vi "bigcryo-T-full_step.vi"() -> (2 "VTI [K]":dbl=99.5, 3 "Spl [K]":dbl=292.757)   [LabVIEW 2019]
uses:
  Components/Global 2.vi
  <vilib>/Analysis/NI_AALPro.lvlib
panel:
  out "Exec T":u32=289
  out "Stable?":bool
  in  "stop":bool
  out "Running Sequence":bool
  out "VTI Rate":dbl=-0.0022185709228587803 format="%#.3g"
  out "Rate":dbl=-0.05046918842629548 format="%#.3g"
  in  "Rate":dbl=0.5
  in  "Reset Graph":bool
  in  "Ramp":bool
  in  "Go To":bool
  in  "Set Temp":dbl=100.0
  out "Range":dbl=5.0
  out "Spl":dbl(slide) scale=0.0..100.0
  out "VTI":dbl(slide)=5.7 scale=0.0..100.0
  out "T":cluster{"X":dbl[], "Y":dbl[]}[](graph)=[{"X"=[16.312679499999998, 16.601001399999998, 16.8885939, 17.146738, 17.4184414, 17.704434499999998, 17.976812, 18.2486923, 18.519247699999998, 18.8086779, 19.0817953, 19.3520784, 19.6253158, 19.913267299999998, 20.186597499999998, 20.457057199999998, 20.7287552, 21.0156451, 21.2713833, 21.5449196, 21.834149999999998, 22.1212511, 22.375041, 22.6487737, 22.93645, 23.2227294, 23.47921, 23.751889799999997, 24.0381173, 24.3104694, 24.5817102, 24.8549242, 25.1436846, 25.4137649, 25.6865617, 25.9587959, 26.2467246, 26.519138299999998, 26.788798399999997, 27.0636323, 27.351064299999997, 27.6211639, 27.894986399999997, 28.1650033, 28.4524293, 28.7077293, 28.981569999999998, 29.2689606, 29.5564118, 29.8125924, 30.0829135, 30.3731589, 30.6605563, 30.9164724, 31.1880325, 31.476441299999998, 31.7628693, 32.0191987, 32.291540399999995, 32.581536899999996, 32.8666054, 33.123576199999995, 33.393609399999995, 33.6835326, 33.9546916, 34.2266786, 34.5016617, 34.7865946, 35.0595013, 35.3305311, 35.6012708, 35.8907765, 36.1449745, 36.4181133, 36.7055869, 36.9932881, 37.2491099, 37.5211332, 37.8092405, 38.096976999999995, 38.3524566, 38.6252108, 38.9137998, 39.202196099999995, 39.4708979, 39.7266816, 40.0164993, 40.2877493, 40.5591022, 40.8298363, 41.1201748, 41.392564, 41.6641809, 41.935850699999996, 42.224531999999996, 42.493339299999995, 42.767248699999996, 43.0566812, 43.341667699999995, 43.6315349, 43.9040886, 44.1748267, 44.461991399999995, 44.7503789, 45.0366612, 45.292437799999995, 45.5670358, 45.8529609, 46.1413034, 46.397208199999994, 46.6697953, 46.955648, 47.2436574, 47.50036, 47.773001099999995, 48.060690199999996, 48.347202599999996, 48.6065446, 48.8750785, 49.1640923, 49.4524638, 49.708949, 49.9802385, 50.266528199999996, 50.5407401, 50.812329999999996, 51.0825536], "Y"=[99.498, 99.498, 99.498, 99.498, 99.498, 99.499, 99.499, 99.499, 99.5, 99.5, 99.5, 99.5, 99.5, 99.5, 99.5, 99.501, 99.501, 99.5, 99.5, 99.501, 99.5, 99.501, 99.501, 99.501, 99.501, 99.501, 99.501, 99.501, 99.501, 99.501, 99.501, 99.5, 99.5, 99.5, 99.5, 99.5, 99.501, 99.501, 99.502, 99.502, 99.502, 99.503, 99.502, 99.503, 99.503, 99.502, 99.502, 99.501, 99.501, 99.501, 99.501, 99.5, 99.499, 99.499, 99.499, 99.499, 99.5, 99.501, 99.501, 99.501, 99.501, 99.5, 99.5, 99.5, 99.501, 99.501, 99.501, 99.501, 99.501, 99.501, 99.5, 99.5, 99.5, 99.5, 99.501, 99.501, 99.501, 99.5, 99.5, 99.5, 99.501, 99.5, 99.5, 99.499, 99.499, 99.499, 99.499, 99.499, 99.499, 99.499, 99.5, 99.499, 99.499, 99.499, 99.499, 99.5, 99.5, 99.5, 99.5, 99.5, 99.5, 99.5, 99.5, 99.501, 99.5, 99.501, 99.5, 99.5, 99.501, 99.5, 99.501, 99.501, 99.502, 99.501, 99.501, 99.501, 99.501, 99.5, 99.501, 99.5, 99.5, 99.5, 99.5, 99.5, 99.499, 99.499, 99.5]}, {"X"=[16.312679499999998, 16.601001399999998, 16.8885939, 17.146738, 17.4184414, 17.704434499999998, 17.976812, 18.2486923, 18.519247699999998, 18.8086779, 19.0817953, 19.3520784, 19.6253158, 19.913267299999998, 20.186597499999998, 20.457057199999998, 20.7287552, 21.0156451, 21.2713833, 21.5449196, 21.834149999999998, 22.1212511, 22.375041, 22.6487737, 22.93645, 23.2227294, 23.47921, 23.751889799999997, 24.0381173, 24.3104694, 24.5817102, 24.8549242, 25.1436846, 25.4137649, 25.6865617, 25.9587959, 26.2467246, 26.519138299999998, 26.788798399999997, 27.0636323, 27.351064299999997, 27.6211639, 27.894986399999997, 28.1650033, 28.4524293, 28.7077293, 28.981569999999998, 29.2689606, 29.5564118, 29.8125924, 30.0829135, 30.3731589, 30.6605563, 30.9164724, 31.1880325, 31.476441299999998, 31.7628693, 32.0191987, 32.291540399999995, 32.581536899999996, 32.8666054, 33.123576199999995, 33.393609399999995, 33.6835326, 33.9546916, 34.2266786, 34.5016617, 34.7865946, 35.0595013, 35.3305311, 35.6012708, 35.8907765, 36.1449745, 36.4181133, 36.7055869, 36.9932881, 37.2491099, 37.5211332, 37.8092405, 38.096976999999995, 38.3524566, 38.6252108, 38.9137998, 39.202196099999995, 39.4708979, 39.7266816, 40.0164993, 40.2877493, 40.5591022, 40.8298363, 41.1201748, 41.392564, 41.6641809, 41.935850699999996, 42.224531999999996, 42.493339299999995, 42.767248699999996, 43.0566812, 43.341667699999995, 43.6315349, 43.9040886, 44.1748267, 44.461991399999995, 44.7503789, 45.0366612, 45.292437799999995, 45.5670358, 45.8529609, 46.1413034, 46.397208199999994, 46.6697953, 46.955648, 47.2436574, 47.50036, 47.773001099999995, 48.060690199999996, 48.347202599999996, 48.6065446, 48.8750785, 49.1640923, 49.4524638, 49.708949, 49.9802385, 50.266528199999996, 50.5407401, 50.812329999999996, 51.0825536], "Y"=[292.743, 292.755, 292.765, 292.763, 292.773, 292.772, 292.766, 292.779, 292.785, 292.778, 292.764, 292.754, 292.748, 292.753, 292.754, 292.771, 292.771, 292.764, 292.753, 292.757, 292.751, 292.75, 292.763, 292.761, 292.764, 292.763, 292.768, 292.761, 292.761, 292.749, 292.776, 292.764, 292.769, 292.772, 292.771, 292.768, 292.772, 292.77, 292.769, 292.764, 292.773, 292.78, 292.785, 292.78, 292.761, 292.76, 292.757, 292.773, 292.779, 292.791, 292.776, 292.776, 292.783, 292.783, 292.776, 292.762, 292.767, 292.778, 292.778, 292.767, 292.765, 292.769, 292.769, 292.773, 292.768, 292.766, 292.761, 292.762, 292.737, 292.748, 292.752, 292.739, 292.739, 292.731, 292.734, 292.746, 292.733, 292.732, 292.727, 292.736, 292.742, 292.736, 292.735, 292.747, 292.766, 292.768, 292.755, 292.749, 292.768, 292.761, 292.772, 292.759, 292.756, 292.759, 292.753, 292.747, 292.751, 292.742, 292.738, 292.746, 292.745, 292.743, 292.744, 292.737, 292.745, 292.757, 292.756, 292.769, 292.753, 292.757, 292.75, 292.751, 292.74, 292.737, 292.748, 292.758, 292.765, 292.765, 292.761, 292.759, 292.757, 292.756, 292.757, 292.754, 292.759, 292.763, 292.757]}] caption="XY Graph"
  out "Set VTI [K]":dbl=99.5
  out "Set Spl [K]":dbl=100.0
  # "Heaters"
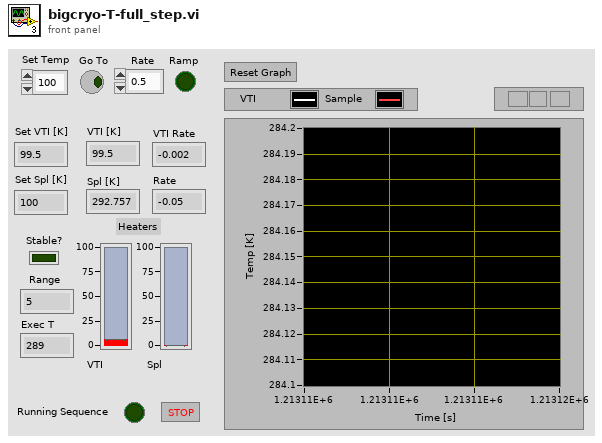
[diagram p1: front panel]
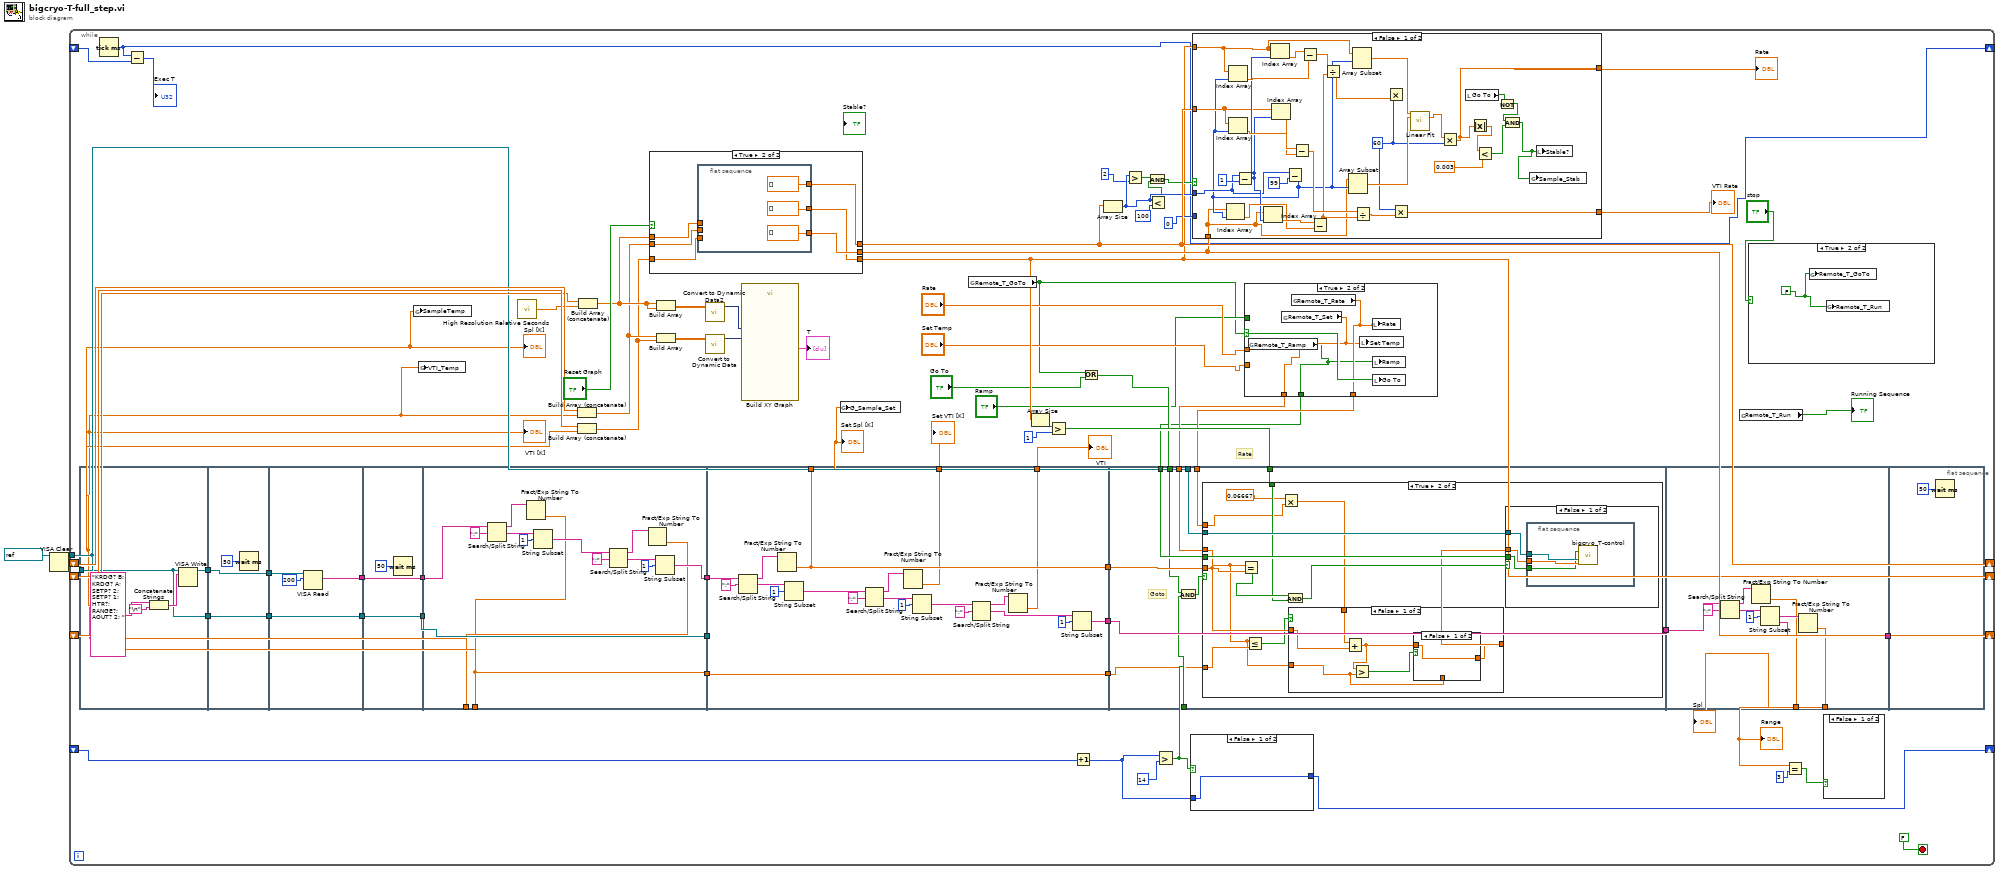
[diagram p0: block diagram]
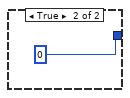
[diagram p2: hidden frame]
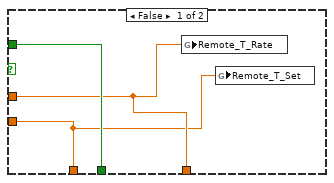
[diagram p4: hidden frame]
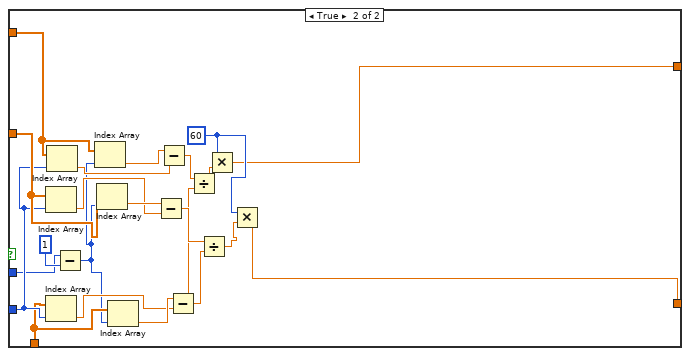
[diagram p5: hidden frame]
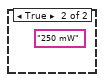
[diagram p7: hidden frame]
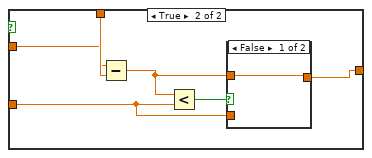
[diagram p10: hidden frame]
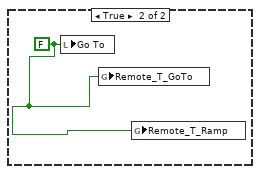
[diagram p12: hidden frame]
diagram:
  n1 = VISA Clear(VISA resource name=refnum<visa-resource-name> "COM7" ("Lakeshore Address")) -> (VISA resource name out=w2:refnum<visa-resource-name>)  [unwired: 1 in, 1 out]
  n2 = while {
    tunnel: w2 -> [w44]
    shift-right: [w29] -> _
    shift-left: _ -> [w72]
    shift-right: [w41] -> _
    shift-left: _ -> [w71]
    shift-right: [w38] -> _
    shift-left: _ -> [w69]
    shift-right: [w15] -> _
    shift-left: _ -> [w17]
    shift-right: [w11] -> _
    shift-left: _ -> [w10]
    stop <- FALSE stop-if-true
    # "Rate"
    n3 = flat-sequence {
      tunnel: w44 -> [w152]
      tunnel: [w152] -> w54
      tunnel: [w151] -> w51
      tunnel: w54 -> [w158]
      tunnel: [w158] -> w53
      tunnel: [w156] -> w52
      tunnel: w51 -> [w156]
      tunnel: [w162] -> w60
      tunnel: w53 -> [w162]
      tunnel: w52 -> [w160]
      tunnel: [w159] -> w48
      tunnel: [w165] -> w76
      tunnel: w60 -> [w165]
      tunnel: [w163] -> w49
      tunnel: w48 -> [w163]
      tunnel: w76 -> [w179]
      tunnel: [w167] -> w6
      tunnel: [w166] -> w7
      tunnel: [w179] -> w73
      tunnel: [w168] -> w50
      tunnel: w49 -> [w170]
      tunnel: [w166] -> w9
      tunnel: [w199] -> w46
      tunnel: [w198] -> w43
      tunnel: [w197] -> w63
      tunnel: [w191] -> w75
      tunnel: [w198] -> w3
      tunnel: w50 -> [w182]
      tunnel: w73 -> [_]
      tunnel: w9 -> [w180]
      tunnel: [w180] -> w8
      tunnel: w46 -> [w210]
      tunnel: [w210] -> w45
      tunnel: w25 -> [w202]
      tunnel: w44 -> [w209]
      tunnel: w21 -> [w208]
      tunnel: w19 -> [w207]
      tunnel: w23 -> [w206]
      tunnel: w43 -> [w205]
      tunnel: w27 -> [w204]
      tunnel: w13 -> [w203]
      tunnel: w8 -> [w200]
      tunnel: [w254] -> w47
      tunnel: [w253] -> w42
      tunnel: w45 -> [w247]
      tunnel: [w252] -> w55
      tunnel: w47 -> [_]
      frame #0 {
        n4 = Concatenate Strings("KRDG? B; KRDG? A; SETP? 2; SETP? 1; HTR?; RANGE?; AOUT? 2; " ("write buffer"), "\n") -> (w153:string)
        n5 = VISA Write(VISA resource name=w152, write buffer=w153) -> (VISA resource name out=w151:refnum<visa-resource-name>)  [unwired: 1 in, 2 out]
      }
      frame #1 {
        n6 = Wait (ms)(milliseconds to wait=50) -> ()  [unwired: 1 out]
      }
      frame #2 {
        n7 = VISA Read(VISA resource name=w160, byte count=u32 200) -> (read buffer=w159:string)  [unwired: 1 in, 3 out]
      }
      frame #3 {
        n8 = Wait (ms)(milliseconds to wait=50) -> ()  [unwired: 1 out]
      }
      frame #4 {
        n9 = Search/Split String(string=w170, search string/char (-)=";") -> (substring before match=w175:string, match + rest of string=w177:string)  [unwired: 1 in, 1 out]
        n10 = Fract/Exp String To Number(string=w175) -> (number=w166:dbl)  [unwired: 3 in, 1 out]
        n11 = String Subset(string=w177, offset (0)=u32 1 ("byte count")) -> (substring=w169:string)  [unwired: 1 in]
        n12 = Search/Split String(string=w169, search string/char (-)=";") -> (substring before match=w171:string, match + rest of string=w173:string)  [unwired: 1 in, 1 out]
        n13 = Fract/Exp String To Number(string=w171) -> (number=w167:dbl)  [unwired: 3 in, 1 out]
        n14 = String Subset(string=w173, offset (0)=u32 1 ("byte count")) -> (substring=w168:string)  [unwired: 1 in]
      }
      frame #5 {
        n15 = Search/Split String(string=w182, search string/char (-)=";") -> (substring before match=w181:string, match + rest of string=w184:string)  [unwired: 1 in, 1 out]
        n16 = Fract/Exp String To Number(string=w181) -> (number=w198:dbl)  [unwired: 3 in, 1 out]
        n17 = String Subset(string=w184, offset (0)=u32 1 ("byte count")) -> (substring=w187:string)  [unwired: 1 in]
        n18 = Search/Split String(string=w187, search string/char (-)=";") -> (substring before match=w186:string, match + rest of string=w189:string)  [unwired: 1 in, 1 out]
        n19 = Fract/Exp String To Number(string=w186) -> (number=w191:dbl)  [unwired: 3 in, 1 out]
        n20 = String Subset(string=w189, offset (0)=u32 1 ("byte count")) -> (substring=w193:string)  [unwired: 1 in]
        n21 = Search/Split String(string=w193, search string/char (-)=";") -> (substring before match=w192:string, match + rest of string=w195:string)  [unwired: 1 in, 1 out]
        n22 = Fract/Exp String To Number(string=w192) -> (number=w197:dbl)  [unwired: 3 in, 1 out]
        n23 = String Subset(string=w195, offset (0)=u32 1 ("byte count")) -> (substring=w199:string)  [unwired: 1 in]
      }
      frame #6 {
        # "Goto"
        n24 = And(x=w202, y=w203) -> (x .and. y?=w201:bool)
        n25 = case shown="True" w201 {
          tunnel: w209 -> [_ w223]
          tunnel: w208 -> [_ w211]
          tunnel: w207 -> [_ w222]
          tunnel: w206 -> [_ w217]
          tunnel: w205 -> [_ w214]
          tunnel: w204 -> [_ w220]
          tunnel: w200 -> [_ w216]
          frame False {
          }
          frame True {
            n26 = Equal?(x=w211, y=w214) -> (x = y?=w221:bool)
            n27 = Less Or Equal?(x=w211, y=w216) -> (x <= y?=w212:bool)
            n28 = Multiply(x=0.06667, y=w217) -> (x*y=w215:dbl)
            n29 = And(x=w221, y=w220) -> (x .and. y?=w219:bool)
            n30 = case shown="False" w212 {
              tunnel: w215 -> [w229 w237]
              tunnel: w214 -> [w228 w236]
              tunnel: [w224 w233] -> w213
              tunnel: w211 -> [w227 w232]
              frame False {
                n31 = Add(x=w229, y=w228) -> (x+y=w225:dbl)
                n32 = Greater?(x=w225, y=w227) -> (0:w226:bool)
                n33 = case shown="False" w226 {
                  tunnel: w227 -> [_ w231]
                  tunnel: w225 -> [w230 _]
                  tunnel: [w230 w231] -> w224
                  frame False {
                  }
                  frame True {
                  }
                }
              }
              frame True {
                n34 = Subtract(x=w236, y=w237) -> (x-y=w234:dbl)
                n35 = Less?(x=w234, y=w232) -> (x < y?=w235:bool)
                n36 = case shown="False" w235 {
                  tunnel: w234 -> [w238 _]
                  tunnel: [w238 w239] -> w233
                  tunnel: w232 -> [_ w239]
                  frame False {
                  }
                  frame True {
                  }
                }
              }
            }
            n37 = case shown="False" w219 {
              tunnel: w223 -> [w242 _]
              tunnel: w213 -> [w241 _]
              tunnel: w222 -> [w240 _]
              frame False {
                n38 = flat-sequence {
                  tunnel: w242 -> [w245]
                  tunnel: w241 -> [w244]
                  tunnel: w240 -> [w243]
                  frame #0 {
                    n39 = call "bigcryo_T-control.vi"("Ramp Mode"=w243, "VISA resource name out"=w245, "Set Sample Temp [K]"=w244) -> ()  [unwired: 13 in]
                  }
                }
              }
              frame True {
                w246 = FALSE
                n40 = local write "Go To"(w246) -> ()
                n41 = global write "Global 2.vi" "Remote_T_GoTo"(w246) -> ()
                n42 = global write "Global 2.vi" "Remote_T_Ramp"(w246) -> ()
              }
            }
          }
        }
      }
      frame #7 {
        n43 = Search/Split String(string=w247, search string/char (-)=";") -> (substring before match=w248:string, match + rest of string=w250:string)  [unwired: 1 in, 1 out]
        n44 = Fract/Exp String To Number(string=w248) -> (number=w252:dbl)  [unwired: 3 in, 1 out]
        n45 = String Subset(string=w250, offset (0)=u32 1 ("byte count")) -> (substring=w254:string)  [unwired: 1 in]
        n46 = Fract/Exp String To Number(string=w254) -> (number=w253:dbl)  [unwired: 3 in, 1 out]
      }
      frame #8 {
        n47 = Wait (ms)(milliseconds to wait=50) -> ()  [unwired: 1 out]
      }
    }
    n48 = Tick Count (ms)() -> (millisecond timer value=w15:u32)
    n49 = Subtract(x=w15, y=w17) -> (x-y=→"Exec T":u32)
    n50 = global write "Global 2.vi" "SampleTemp"(w7) -> ()
    n51 = global write "Global 2.vi" "VTI_Temp"(w6) -> ()
    n52 = call <vilib>:"High Resolution Relative Seconds.vi"() -> ("relative seconds"=w68:dbl)
    n53 = Build Array (concatenate)(w71, w6) -> (w57:dbl[])
    n54 = Build Array (concatenate)(w72, w7) -> (w56:dbl[])
    n55 = Build Array (concatenate)(w69, w68) -> (w58:dbl[])
    n56 = case shown="True" "Reset Graph" {
      tunnel: w58 -> [w141 w147]
      tunnel: [w141 w146] -> w38
      tunnel: w57 -> [w140 w145]
      tunnel: [w140 w144] -> w41
      tunnel: w56 -> [w139 w143]
      tunnel: [w139 w142] -> w29
      frame False {
      }
      frame True {
        n57 = flat-sequence {
          tunnel: w147 -> [_]
          tunnel: w145 -> [_]
          tunnel: w143 -> [_]
          tunnel: [dbl[] []] -> w144
          tunnel: [dbl[] []] -> w146
          tunnel: [dbl[] []] -> w142
          frame #0 {
          }
        }
      }
    }
    n58 = Build Array(w58, w58) -> (w65:dbl[][])
    n59 = Build Array(w57, w56) -> (w67:dbl[][])
    n60 = call "Convert to Dynamic Data2"("2D Array"=w65) -> ("Dynamic Data Type"=w64:dynamicdata)  [unwired: 3 in]
    n61 = call "Convert to Dynamic Data"("2D Array"=w67) -> ("Dynamic Data Type"=w66:dynamicdata)  [unwired: 3 in]
    n62 = call "Build XY Graph"("Y Input"=w66, "X Input"=w64) -> ("XY Graph"=→"T":cluster{"X":dbl[], "Y":dbl[]}[])  [unwired: 8 in, 1 out]
    n63 = global write "Global 2.vi" "G_Sample_Set"(w3) -> ()
    n64 = global read "Global 2.vi" "Remote_T_GoTo"() -> (w5:bool)
    n65 = Array Size(array=w29) -> (size(s)=w30:i32)
    n66 = Greater?(x=w30, y=1) -> (0:w27:bool)
    n67 = Increment(x=w10) -> (x+1=w12:i32)
    n68 = Or(x=w5, y="Go To") -> (x .or. y?=w25:bool)
    n69 = Array Size(array=w41) -> (size(s)=w35:i32)
    n70 = Greater?(x=w35, y=2) -> (0:w37:bool)
    n71 = Less?(x=w35, y=100) -> (x < y?=w33:bool)
    n72 = And(x=w37, y=w33) -> (x .and. y?=w36:bool)
    n73 = Greater?(x=w12, y=14) -> (0:w13:bool)
    n74 = case shown="False" w13 {
      tunnel: [w77 0] -> w11
      tunnel: w12 -> [w77 _]
      frame False {
      }
      frame True {
      }
    }
    n75 = case shown="False" w36 {
      tunnel: w41 -> [w101 w138]
      tunnel: 0 -> [_ w137]
      tunnel: w35 -> [w103 w121]
      tunnel: w38 -> [w98 w135]
      tunnel: w29 -> [w100 w136]
      tunnel: [w92 w119] -> w32
      tunnel: [w104 w118] -> w31
      frame False {
        w95 = 60
        n76 = Subtract(x=w103, y=1) -> (x-y=w105:i32)
        n77 = Index Array(array=w98, index=w105) -> (element=w117:dbl)
        n78 = Index Array(array=w100, index=w105) -> (element=w113:dbl)
        n79 = Index Array(array=w101, index=w105) -> (element=w115:dbl)
        n80 = Subtract(x=w103, y=99) -> (x-y=w99:i32)
        n81 = Index Array(array=w98, index=w99) -> (element=w116:dbl)
        n82 = Index Array(array=w100, index=w99) -> (element=w112:dbl)
        n83 = Index Array(array=w101, index=w99) -> (element=w114:dbl)
        n84 = Subtract(x=w115, y=w114) -> (x-y=w110:dbl)
        n85 = Subtract(x=w113, y=w112) -> (x-y=w111:dbl)
        n86 = Subtract(x=w117, y=w116) -> (x-y=w109:dbl)
        n87 = Divide(x=w111, y=w109) -> (x/y=w108:dbl)
        n88 = Array Subset(array=w98, index=w99) -> (w96:dbl[])  [unwired: 1 in]
        n89 = Array Subset(array=w100, index=w99) -> (w97:dbl[])  [unwired: 1 in]
        n90 = Divide(x=w110, y=w109) -> (x/y=w107:dbl)
        n91 = Multiply(x=w95, y=w108) -> ()  [unwired: 1 out]
        n92 = Multiply(x=w95, y=w107) -> (x*y=w104:dbl)
        n93 = call <vilib>:"Linear Fit.vi"("Y"=w97, "X"=w96) -> ("slope"=w94:dbl)  [unwired: 9 in, 4 out]
        n94 = Multiply(x=w94, y=w95) -> (x*y=w92:dbl)
        n95 = local read "Go To"() -> (w89:bool)
        n96 = Absolute Value(x=w92) -> (abs(x)=w91:dbl)
        n97 = Less?(x=w91, y=0.003) -> (x < y?=w90:bool)
        n98 = Not(x=w89) -> (.not. x?=w88:bool)
        n99 = And(x=w88, y=w90) -> (x .and. y?=w87:bool)
        n100 = global write "Global 2.vi" "Sample_Stab"(w87) -> ()
        n101 = local write "Stable?"(w87) -> ()
      }
      frame True {
        w124 = 60
        n102 = Index Array(array=w138, index=w137) -> (element=w131:dbl)
        n103 = Index Array(array=w135, index=w137) -> (element=w133:dbl)
        n104 = Index Array(array=w136, index=w137) -> (element=w129:dbl)
        n105 = Subtract(x=w121, y=1) -> (x-y=w120:i32)
        n106 = Index Array(array=w136, index=w120) -> (element=w130:dbl)
        n107 = Index Array(array=w138, index=w120) -> (element=w132:dbl)
        n108 = Index Array(array=w135, index=w120) -> (element=w134:dbl)
        n109 = Subtract(x=w132, y=w131) -> (x-y=w127:dbl)
        n110 = Subtract(x=w130, y=w129) -> (x-y=w128:dbl)
        n111 = Subtract(x=w134, y=w133) -> (x-y=w126:dbl)
        n112 = Divide(x=w128, y=w126) -> (x/y=w125:dbl)
        n113 = Divide(x=w127, y=w126) -> (x/y=w123:dbl)
        n114 = Multiply(x=w124, y=w125) -> (x*y=w119:dbl)
        n115 = Multiply(x=w124, y=w123) -> (x*y=w118:dbl)
      }
    }
    "Rate" <- w32
    "VTI Rate" <- w31
    n116 = case shown="True" w5 {
      selector: w5 -> [_ w86]
      tunnel: "Rate" -> [w81 _]
      tunnel: [w81 w85] -> w23
      tunnel: "Set Temp" -> [w80 _]
      tunnel: [w80 w84] -> w21
      tunnel: "Ramp" -> [w82 _]
      tunnel: [w82 w83] -> w19
      frame False {
        n117 = global write "Global 2.vi" "Remote_T_Rate"(w81) -> ()
        n118 = global write "Global 2.vi" "Remote_T_Set"(w80) -> ()
      }
      frame True {
        n119 = global read "Global 2.vi" "Remote_T_Ramp"() -> (w83:bool)
        n120 = global read "Global 2.vi" "Remote_T_Set"() -> (w84:dbl)
        n121 = global read "Global 2.vi" "Remote_T_Rate"() -> (w85:dbl)
        n122 = local write "Set Temp"(w84) -> ()
        n123 = local write "Rate"(w85) -> ()
        n124 = local write "Ramp"(w83) -> ()
        n125 = local write "Go To"(w86) -> ()
      }
    }
    n126 = global read "Global 2.vi" "Remote_T_Run"() -> (→"Running Sequence":bool)
    n127 = case shown="True" "stop" {
      frame False {
      }
      frame True {
        w79 = FALSE
        n128 = global write "Global 2.vi" "Remote_T_GoTo"(w79) -> ()
        n129 = global write "Global 2.vi" "Remote_T_Run"(w79) -> ()
      }
    }
    n130 = Equal?(x=w55, y=3) -> (x = y?=w61:bool)
    n131 = case shown="False" w61 {
      frame False {
      }
      frame True {
        (unwired) "250 mW"
      }
    }
    "Spl [K]" <- w7
    "VTI [K]" <- w6
    "Set Spl [K]" <- w3
    "Set VTI [K]" <- w75
    "VTI" <- w63
    "Spl" <- w42
    "Range" <- w55
  }
